vi "Base_eleve.vi"() -> ()   [LabVIEW 2018]
uses:
  <vilib>/Instr/_visa.llb/VISA Configure Serial Port (Instr).vi
panel:
  in  "Pause/Go":bool
  out "Humidity Chart":dbl(graph)
  out "Pressure Chart":dbl(graph)
  out "Temperature Chart":dbl(graph)
  out "Humidity":dbl
  out "Pressure":dbl
  out "Temperature":dbl
  out "Chaîne":string
  in  "stop":bool
  in  "Nom de ressource VISA":refnum<visa-resource-name>
  # "1. Brancher la carte Arduino sur un port USB\n2. Choisir le port COM de la carte dans la liste déroulante \"Nom de ressource VISA\"\n3. Lancer le programme"
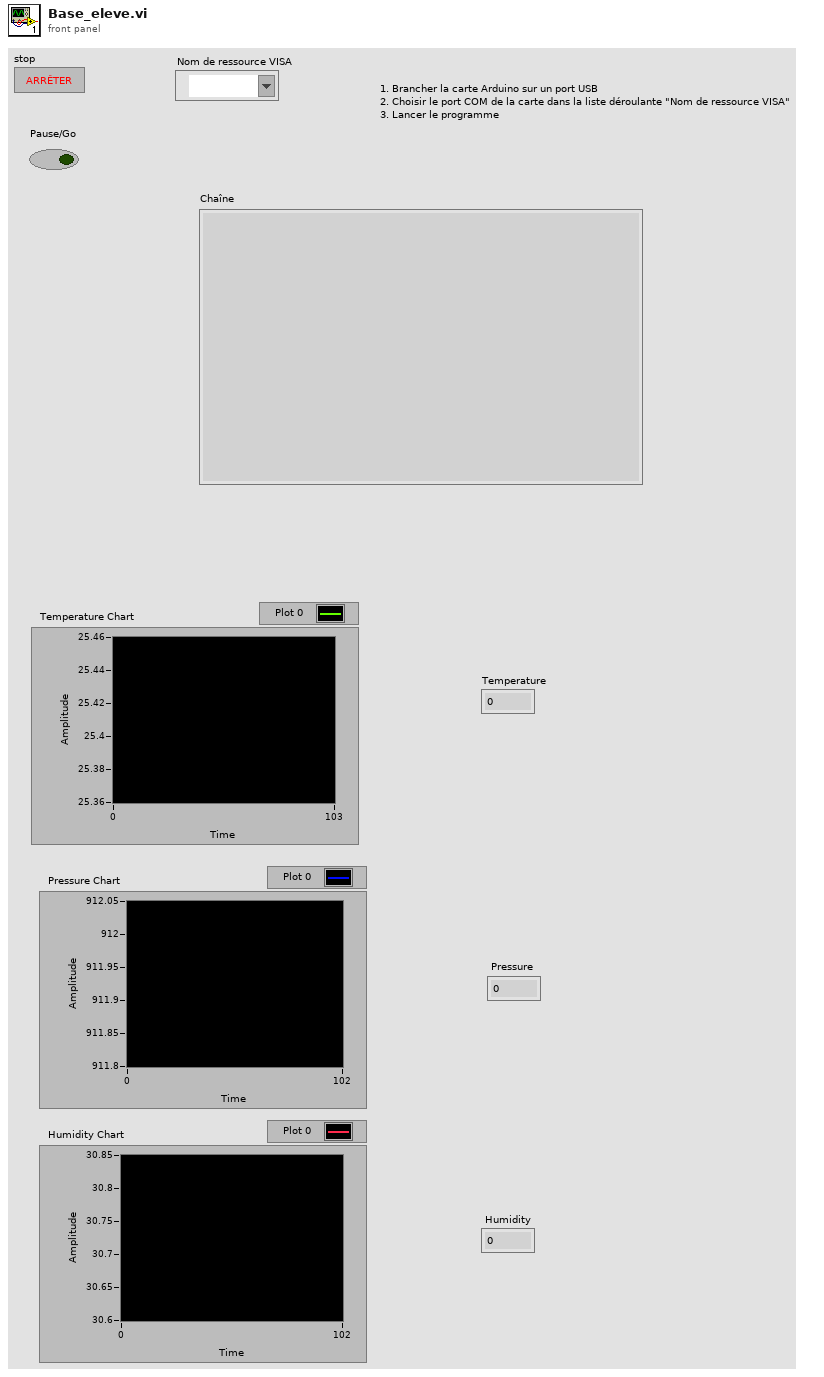
[diagram p1: front panel]
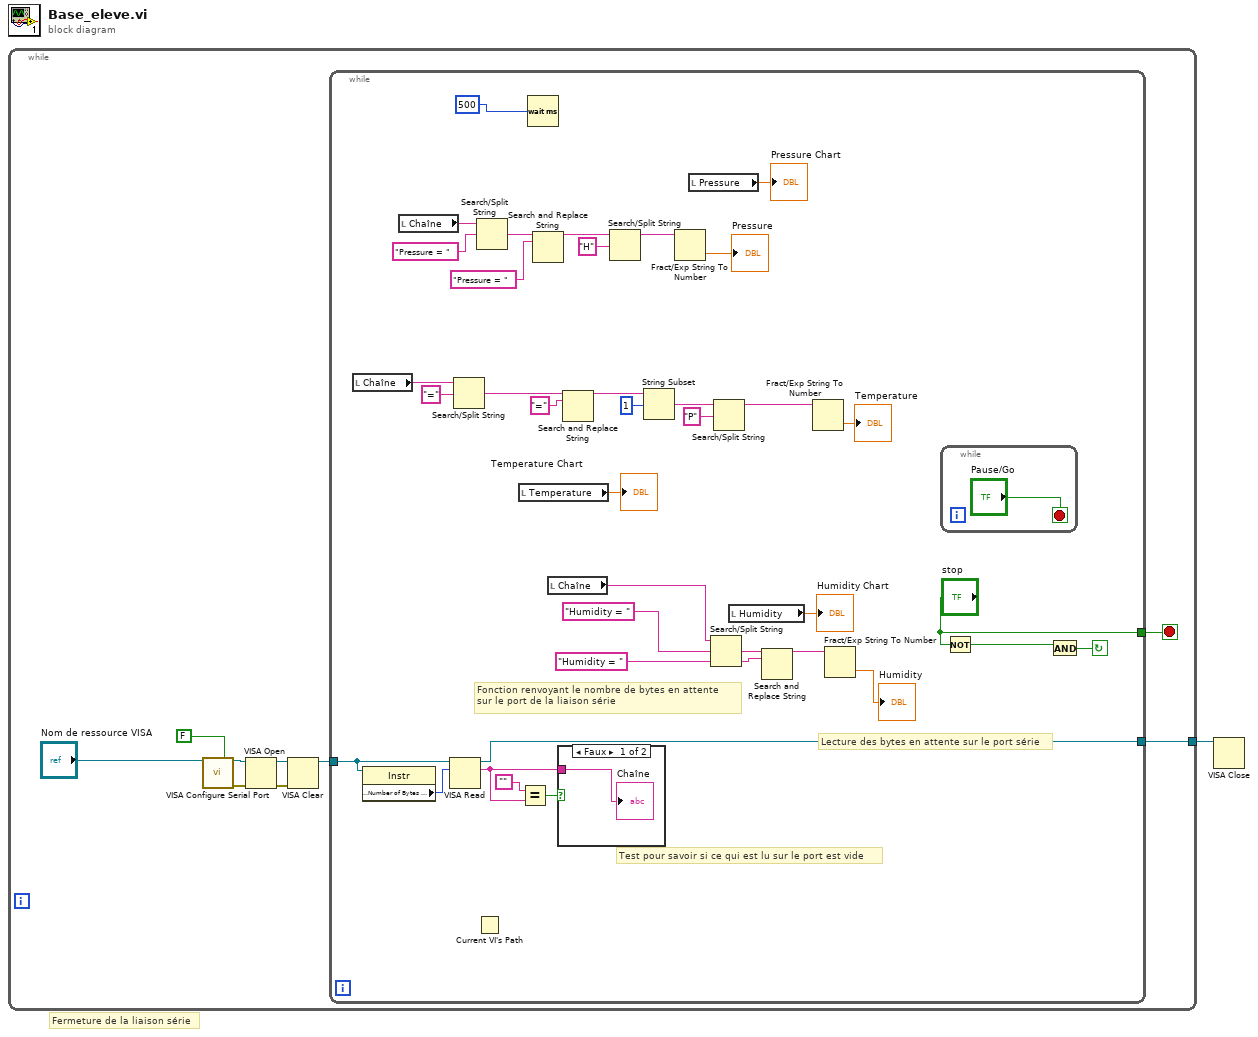
[diagram p0: block diagram]
diagram:
  # "Fermeture de la liaison série"
  n1 = while {
    tunnel: [w2] -> w1
    stop <- w3 stop-if-true
    n2 = call-poly "VISA Configure Serial Port"("VISA resource name"="Nom de ressource VISA", "Enable Termination\nChar (T)"=FALSE ("Enable Termination\nChar (T)")) -> ("VISA resource name out"=w8:refnum<visa-resource-name>, "error out"=w9:errorcluster)  [unwired: 12 in]
    n3 = VISA Open(error in (no error)=w9, VISA resource name=w8) -> (VISA resource name=w6:refnum<visa-resource-name>, error out=w10:errorcluster)  [unwired: 3 in]
    n4 = VISA Clear(VISA resource name=w6, error in (no error)=w10) -> (VISA resource name out=w7:refnum<visa-resource-name>)  [unwired: 1 out]
    n5 = while {
      tunnel: w7 -> [w47]
      tunnel: [w45] -> w2
      tunnel: ["stop"] -> w3
      stop <- w40 continue-if-true
      # "Lecture des bytes en attente sur le port série"
      # "Fonction renvoyant le nombre de bytes en attente\nsur le port de la liaison série"
      # "Test pour savoir si ce qui est lu sur le port est vide"
      n6 = local read "Chaîne"() -> (w31:string)
      n7 = property class="Instr"(reference=w47) -> ("Serial Settings:Number of Bytes at Serial Port"=w46:u32)  [unwired: 1 in, 2 out]
      n8 = local read "Chaîne"() -> (w20:string)
      n9 = VISA Read(VISA resource name=w47, byte count=w46) -> (VISA resource name out=w45:refnum<visa-resource-name>, read buffer=w42:string)  [unwired: 1 in, 2 out]
      n10 = Search/Split String(string=w31, search string/char (-)="=") -> (match + rest of string=w30:string)  [unwired: 1 in, 2 out]
      n11 = Current VI's Path() -> ()  [unwired: 1 out]
      n12 = Search/Split String(string=w20, search string/char (-)="Pressure = ") -> (match + rest of string=w19:string)  [unwired: 1 in, 2 out]
      n13 = local read "Temperature"() -> (→"Temperature Chart":dbl)
      n14 = Equal?(x="", y=w42) -> (x = y?=w43:bool)
      n15 = Wait (ms)(milliseconds to wait=500) -> ()  [unwired: 1 out]
      n16 = Search and Replace String(input string=w19, search string="Pressure = ") -> (result string=w18:string)  [unwired: 6 in, 3 out]
      n17 = local read "Chaîne"() -> (w37:string)
      n18 = case shown="Faux" w43 {
        tunnel: w42 -> [w49 _]
        frame False {
          "Chaîne" <- w49
        }
        frame True {
        }
      }
      n19 = Search and Replace String(input string=w30, search string="=") -> (result string=w29:string)  [unwired: 6 in, 3 out]
      n20 = Search/Split String(string=w18, search string/char (-)="H") -> (substring before match=w17:string)  [unwired: 1 in, 2 out]
      n21 = String Subset(string=w29, offset (0)=1) -> (substring=w28:string)  [unwired: 1 in]
      n22 = Fract/Exp String To Number(string=w17) -> (number=→"Pressure":dbl)  [unwired: 3 in, 1 out]
      n23 = local read "Pressure"() -> (→"Pressure Chart":dbl)
      n24 = Search/Split String(string=w37, search string/char (-)="Humidity = ") -> (match + rest of string=w38:string)  [unwired: 1 in, 2 out]
      n25 = Search/Split String(string=w28, search string/char (-)="P") -> (substring before match=w27:string)  [unwired: 1 in, 2 out]
      n26 = local read "Humidity"() -> (→"Humidity Chart":dbl)
      n27 = Search and Replace String(input string=w38, search string="Humidity = ") -> (result string=w36:string)  [unwired: 6 in, 3 out]
      n28 = Fract/Exp String To Number(string=w27) -> (number=→"Temperature":dbl)  [unwired: 3 in, 1 out]
      n29 = Fract/Exp String To Number(string=w36) -> (number=→"Humidity":dbl)  [unwired: 3 in, 1 out]
      n30 = while {
        stop <- "Pause/Go" stop-if-true
      }
      n31 = Not(x="stop") -> (.not. x?=w39:bool)
      n32 = And(x=w39) -> (x .and. y?=w40:bool)  [unwired: 1 in]
    }
  }
  n33 = VISA Close(VISA resource name=w1) -> ()  [unwired: 1 in, 1 out]
